vi "ReadAs Stream_Status.vi"(7 "DownloadStats In":T1, 8 "error in (no error)":errorcluster, 11 "HttpContent in":refnum<class "HttpContent.lvclass">) -> (0 "error out":errorcluster, 1 "Length":i64, 2 "Position":i64, 3 "HttpContent out":refnum<class "HttpContent.lvclass">, 4 "Progress":dbl, 5 "RunningStats Out":T1, 6 "Done or Error":bool)   [LabVIEW 2018, in "HttpClient_NET.lvlib" / "HttpContent.lvclass"]
doc: "<b> </b> <b> </b>\nHttpClient_NET\nJustin Young - Viviota\nCopyright (c) 2021\nLicense: BSD"
uses:
  HttpContent.lvclass
  Types/DownloadStats_Cluster.ctl
  HttpContent.lvclass/HttpContent.ctl
  Accessors/Read NET_DestinationStream.vi
  HttpHeaders_content/HttpHeaders_Content.lvclass
  C:/Viviota/Projects/R&D/LabVIEW_HTTP_REST_NET/HTTPHeaders_NET/HttpHeaders_NET.lvclass
  HTTPHeaders_NET/HttpHeaders_NET.lvclass
  HttpClient_NET.lvlib
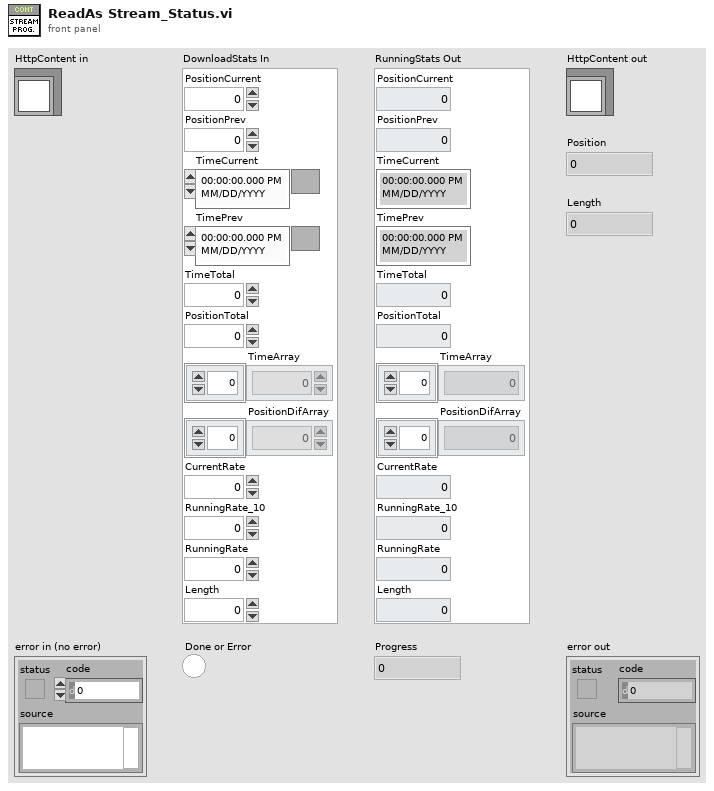
[diagram p1: front panel]
types:
  T1 = typedef "HttpClient_NET.lvlib/DownloadStats_Cluster.ctl" = cluster{"PositionCurrent":dbl, "PositionPrev":dbl, "TimeCurrent":timestamp, "TimePrev":timestamp, "TimeTotal":dbl, "PositionTotal":dbl, "TimeArray":dbl[], "PositionDifArray":dbl[], "CurrentRate":dbl, "RunningRate_10":dbl, "RunningRate":dbl, "Length":dbl}
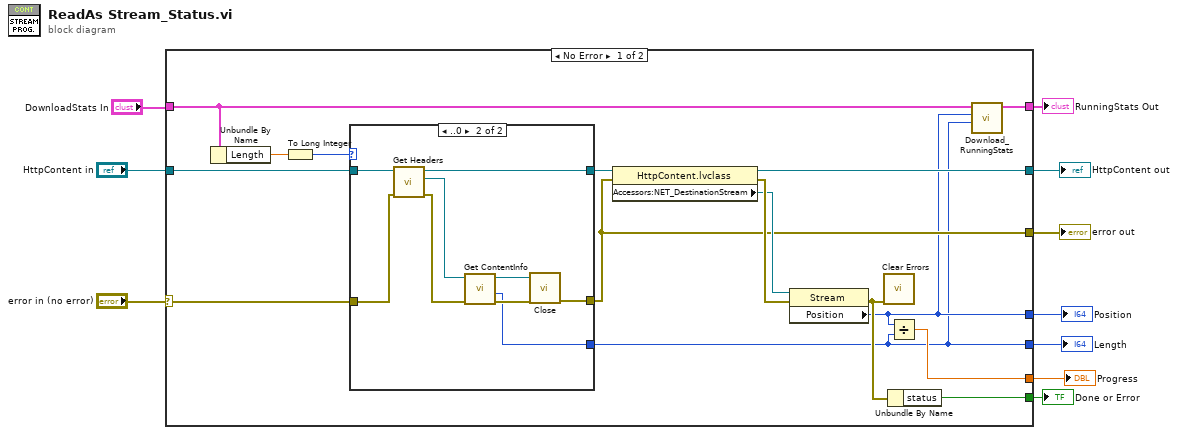
[diagram p0: block diagram]
diagram:
  n1 = case shown="No Error" "error in (no error)" {
    selector: "error in (no error)" -> [w25 w40]
    tunnel: [w26 w41] -> w10
    tunnel: "HttpContent in" -> [w17 w41]
    tunnel: [w20 w40] -> w7
    tunnel: [w15 _] -> w6
    tunnel: [w14 _] -> w5
    tunnel: [w21 _] -> w4
    tunnel: [w18 _] -> w3
    tunnel: "DownloadStats In" -> [w13 w39]
    tunnel: [w16 w39] -> w1
    frame No Error {
      n2 = Unbundle By Name(w13) -> ("Length"=w12:dbl)
      n3 = To Long Integer(number=w12) -> (32bit integer=w11:i32)
      n4 = case shown="..0" w11 {
        selector: w11 -> [w27 _]
        tunnel: w25 -> [w28 w38]
        tunnel: w17 -> [w29 w37]
        tunnel: [w29 w36] -> w24
        tunnel: [w27 w30] -> w14
        tunnel: [w28 w31] -> w20
        frame 1, Default {
        }
        frame ..0 {
          n5 = call "Get Headers.vi"("error in (no error)"=w38, "HttpContent in"=w37) -> ("error out"=w34:errorcluster, "HTTPHeaders"=w35:refnum<class "HttpHeaders_Content.lvclass">, "HttpContent out"=w36:refnum<class "HttpContent.lvclass">)  [unwired: 7 in]
          n6 = call "Get ContentInfo.vi"("error in (no error)"=w34, "HttpHeaders_Content in"=w35) -> ("error out"=w33:errorcluster, "Length"=w30:i64, "HttpHeaders_Content out"=w32:refnum<class "HttpHeaders_Content.lvclass">)  [unwired: 6 in, 1 out]
          n7 = call "Close.vi"("error in (no error)"=w33, "HTTPHeaders_NET in"=w32) -> ("error out"=w31:errorcluster)  [unwired: 9 in]
        }
      }
      n8 = property class="HttpContent.lvclass"(reference=w24, error in=w20) -> (reference out=w26:refnum<class "HttpContent.lvclass">, error out=w23:errorcluster, "Accessors:NET_DestinationStream"=w22:refnum<k24>)
      n9 = property class="Stream"(reference=w22, error in=w23) -> (error out=w19:errorcluster, "Position"=w15:i64)  [unwired: 1 out]
      n10 = call <vilib>:"Clear Errors.vi"("error in (no error)"=w19) -> ()  [unwired: 5 in, 2 out]
      n11 = Unbundle By Name(w19) -> ("status"=w18:bool)
      n12 = Divide(x=w15, y=w14) -> (x/y=w21:dbl)
      n13 = call "Download_RunningStats.vi"("Length"=w14, "Position"=w15, "DownloadStats In"=w13) -> ("RunningStats"=w16:T1)  [unwired: 8 in]
    }
    frame Error {
    }
  }
  "error out" <- w7
  "HttpContent out" <- w10
  "Length" <- w5
  "Position" <- w6
  "Progress" <- w4
  "Done or Error" <- w3
  "RunningStats Out" <- w1
